vi "TimeForSweepRecord.vi"(11 "Time":string) -> (3 "Time representation":i32)   [LabVIEW 2018]
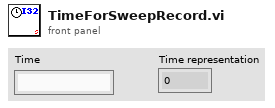
[diagram p1: front panel]
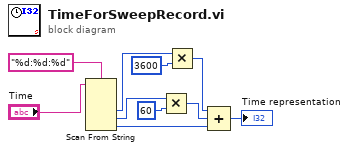
[diagram p0: block diagram]
diagram:
  n1 = Scan From String(format string="%d:%d:%d", input string="Time") -> (output 1=w7:i32, output 2=w4:i32, output 3=w1:i32)  [unwired: 5 in, 3 out]
  n2 = Multiply(x=w4, y=60) -> (x*y=w2:i32)
  n3 = Multiply(x=w7, y=3600) -> (x*y=w3:i32)
  n4 = Compound Arithmetic op=ADD(w3, w2, w1) -> (→"Time representation":i32)
